vi "三段比较器（U32).vi"(1 "低":u32, 2 "输入数值":u32=50, 3 "高":u32=100) -> (0 "Range":enum16{"超低", "适中", "超高"}(ring)=enum."超高")   [LabVIEW 2013]
doc: "功能：\n\n返回一个枚举，表明输入数的范围，用于三段比较。\n\n\nCSXCS_366创建。"
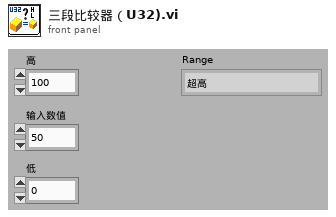
[diagram p1: front panel]
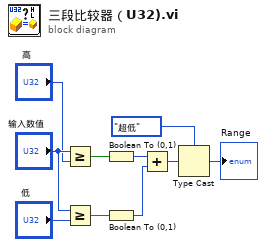
[diagram p0: block diagram]
diagram:
  n1 = Greater Or Equal?(x="输入数值", y="高") -> (x >= y?=w6:bool)
  n2 = Greater Or Equal?(x="输入数值", y="低") -> (x >= y?=w9:bool)
  n3 = Boolean To (0,1)(Boolean=w6) -> (0, 1=w4:i16)
  n4 = Boolean To (0,1)(Boolean=w9) -> (0, 1=w5:i16)
  n5 = Add(x=w4, y=w5) -> (x+y=w3:i16)
  n6 = Type Cast(type=enum16{"超低", "适中", "超高"}."超低" ("Range"), x=w3) -> (*(type *) &x=→"Range":enum16{"超低", "适中", "超高"})
